vi "Get_Delays.vi"(6 "Coincidence Window":dbl, 7 "Coincidences In":u32, 9 "Expected Delay":dbl, 10 "Delay":dbl, 11 "Delays In":dbl[](array[numeric])) -> (1 "Is Coincidence?":bool, 2 "Coincidences out":u32, 3 "Delays Out":dbl[](array[numeric]))   [LabVIEW 2023]
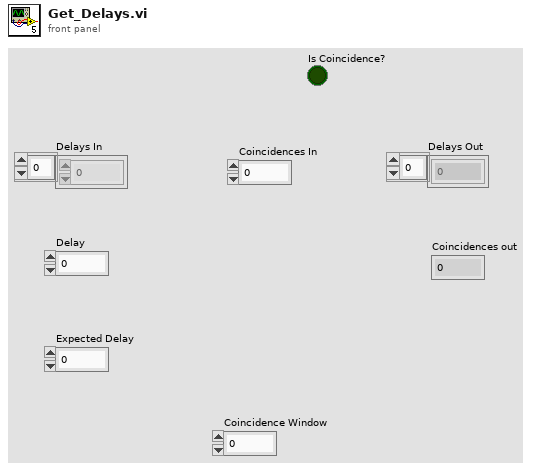
[diagram p1: front panel]
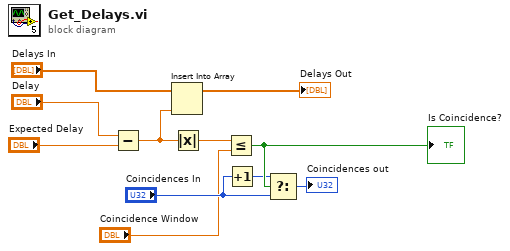
[diagram p0: block diagram]
diagram:
  n1 = Subtract(x="Delay", y="Expected Delay") -> (x-y=w5:dbl)
  n2 = Insert Into Array(array="Delays In", new element=w5) -> (→"Delays Out":dbl[])  [unwired: 1 in]
  n3 = Absolute Value(x=w5) -> (abs(x)=w6:dbl)
  n4 = Less Or Equal?(x=w6, y="Coincidence Window") -> (x <= y?=w9:bool)
  "Is Coincidence?" <- w9
  n5 = Increment(x="Coincidences In") -> (x+1=w8:u32)
  n6 = Select(t=w8, s=w9, f="Coincidences In") -> (s? t:f=→"Coincidences out":u32)
